vi "getType_unused.vi"(8 "error in (no error)":errorcluster, 11 "Control in":refnum<class "Control.lvclass">) -> (0 "error out":errorcluster, 2 "type":refnum<vi>, 3 "Control out":refnum<class "Control.lvclass">)   [LabVIEW 2023]
uses:
  Control.lvclass/Control.ctl
  Control.lvclass
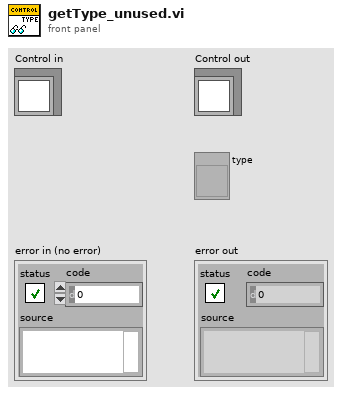
[diagram p1: front panel]
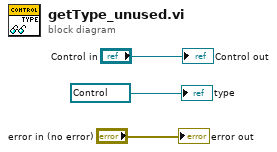
[diagram p0: block diagram]
diagram:
  "error out" <- "error in (no error)"
  "Control out" <- "Control in"
  "type" <- refnum<vi> refnum ("type")
